vi "Sound Play Tone.vi"(5 "device ID":u32, 6 "stop":bool, 7 "Wait":bool=TRUE, 8 "error in":errorcluster, 9 "volume":dbl=100.0, 10 "sample duration (s)":dbl=0.25, 11 "frequency":dbl=440.0 format="%0.2p") -> (0 "error out":errorcluster, 4 "stopped":bool)   [LabVIEW 2018]
doc: "Plays a tone on an audio device.\n\nThe <b>wait</b> input causes this VI to block until the audio card has played all generated samples, so the execution time of the VI will be at least <b>sample duration(s)</b> long. Setting <b>wait</b> to false will cause the VI to return immediately; if used in an untimed loop, it will consume 100% resources. Set <b>wait</b> to true and use in an untimed loop to generate continuous output without overutilizing CPU resources.\n\nThis VI is written like an express VI: references and tasks are opened on first call, sound is output on every call (unless output fails), and the stop input closes all tasks. Use the stopped output to wire into the conditional terminal of a loop."
uses:
  <vilib>/sound2/lvsound2.llb/Sampling Mode.ctl
  <vilib>/sound2/lvsound2.llb/Sound Output Set Volume (Single).vi
  <vilib>/sound2/lvsound2.llb/Sound Output Write (DBL Single).vi
  <vilib>/measure/NI_MABase.lvlib
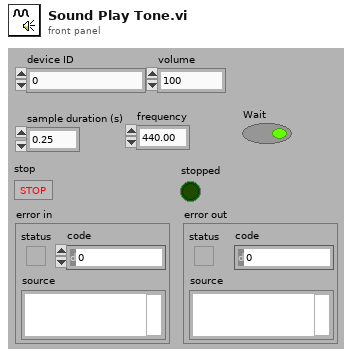
[diagram p1: front panel]
types:
  T1 = typedef "Sampling Mode.ctl" = i32
  T2 = cluster{"Sample Rate":dbl, "nChannels":i32, "Bits per Channel":i32}
  T3 = typedef "Sound Output Task ID.ctl" = u32
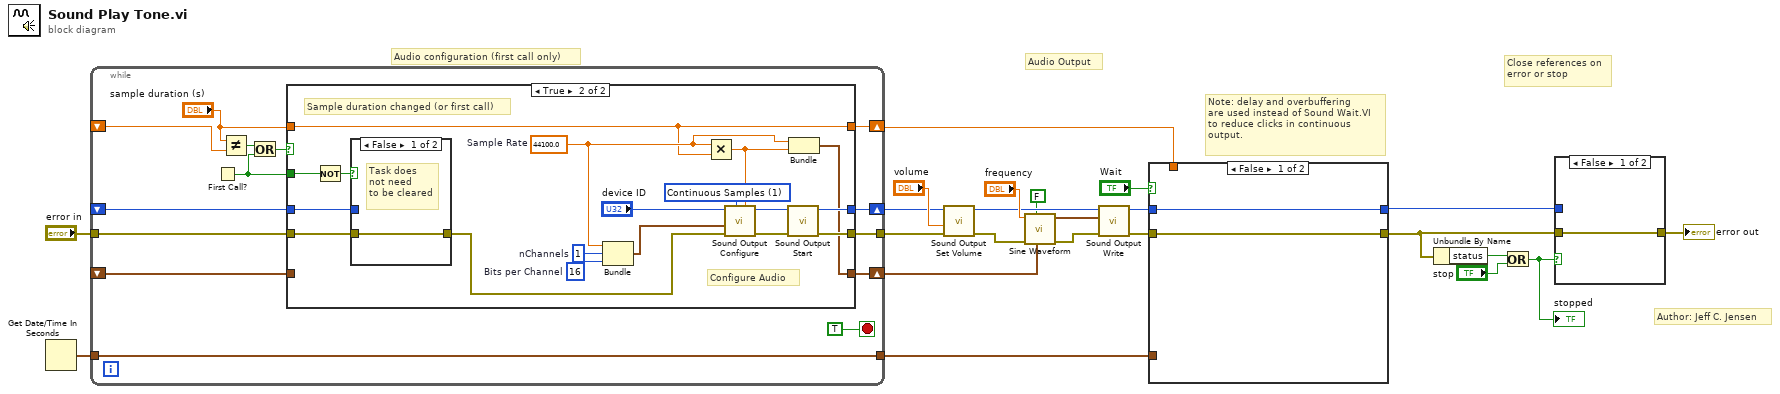
[diagram p0: block diagram]
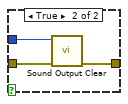
[diagram p2: hidden frame]
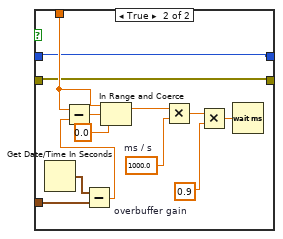
[diagram p3: hidden frame]
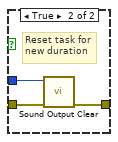
[diagram p5: hidden frame]
diagram:
  # "Note: delay and overbuffering\nare used instead of Sound Wait.VI\nto reduce clicks in continuous\noutput."
  # "Close references on\nerror or stop"
  # "Audio Output"
  # "Author: Jeff C. Jensen"
  # "Audio configuration (first call only)"
  n1 = Get Date/Time In Seconds() -> (seconds since 1Jan1904=w3:timestamp)
  n2 = while {
    tunnel: "error in" -> [w33]
    tunnel: [w37] -> w22
    shift-right: [w35] -> w5
    shift-left: _ -> [w32]
    shift-right: [w34] -> w4
    shift-left: _ -> [w31]
    shift-right: [w30] -> w1
    shift-left: _ -> [w26]
    tunnel: [w24] -> w2
    tunnel: w3 -> [w24]
    stop <- TRUE stop-if-true
    n3 = First Call?() -> (First Call?: T/F=w27:bool)
    n4 = Not Equal?(x="sample duration (s)", y=w26) -> (x != y?=w28:bool)
    n5 = Or(x=w28, y=w27) -> (x .or. y?=w29:bool)
    n6 = case shown="True" w29 {
      tunnel: [w39 w59] -> w37
      tunnel: [w41 w58] -> w35
      tunnel: [w40 w49] -> w34
      tunnel: w33 -> [w39 w46]
      tunnel: w32 -> [w41 w47]
      tunnel: w31 -> [w40 _]
      tunnel: [w38 w42] -> w30
      tunnel: "sample duration (s)" -> [w38 w42]
      tunnel: w27 -> [_ w43]
      frame False {
        # "Audio task already configured."
      }
      frame True {
        w53 = T1 1 items=["Finite Samples", "Continuous Samples"] ("sample mode")
        w48 = 44100.0  # Sample Rate
        w54 = 16  # Bits per Channel
        w55 = 1  # nChannels
        # "Sample duration changed (or first call)"
        # "Configure Audio"
        n7 = Not(x=w43) -> (.not. x?=w45:bool)
        n8 = case shown="False" w45 {
          tunnel: w47 -> [_ w63]
          tunnel: w46 -> [w60 w62]
          tunnel: [w60 w61] -> w44
          frame False {
            # "Task does\nnot need\nto be cleared"
          }
          frame True {
            # "Reset task for\nnew duration"
            n9 = call <vilib>:"Sound Output Clear.vi"("error in (no error)"=w62, "task ID"=w63) -> ("error out"=w61:errorcluster)  [unwired: 9 in]
          }
        }
        n10 = Bundle("Sample Rate"=w48, "nChannels"=w55, "Bits per Channel"=w54) -> (w56:T2)  [unwired: 1 in]
        n11 = Multiply(x=w48, y=w42) -> (x*y=w52:dbl)
        n12 = call <vilib>:"Sound Output Configure.vi"("number of samples/ch"=w52, "sample mode"=w53, "error in (no error)"=w44, "sound format"=w56, "device ID"="device ID") -> ("error out"=w51:errorcluster, "task ID"=w50:T3)  [unwired: 5 in]
        n13 = call <vilib>:"Sound Output Start.vi"("error in (no error)"=w51, "task ID"=w50) -> ("error out"=w59:errorcluster, "task ID out"=w58:T3)  [unwired: 8 in]
        n14 = Bundle("Sample Rate"=w48, w52) -> (w49:cluster{"Sample Rate":dbl, dbl})  [unwired: 1 in]
      }
    }
  }
  n15 = call-poly <vilib>:"Sound Output Set Volume.vi"("error in (no error)"=w22, "volume"="volume", "task ID"=w5) -> ("error out"=w20:errorcluster, "task ID out"=w18:T3)  [unwired: 7 in]
  n16 = call <vilib>:"Sine Waveform.vi"("sampling info"=w4, "reset signal"=FALSE, "error in (no error)"=w20, "frequency"="frequency") -> ("error out"=w17:errorcluster, "signal out"=w16:waveform(dbl))  [unwired: 6 in]
  n17 = call-poly <vilib>:"Sound Output Write.vi"("error in (no error)"=w17, "data"=w16, "task ID"=w18) -> ("error out"=w14:errorcluster, "task ID out"=w15:T3)  [unwired: 7 in]
  n18 = case shown="False" "Wait" {
    tunnel: w15 -> [w65 w70]
    tunnel: w14 -> [w64 w69]
    tunnel: [w64 w69] -> w8
    tunnel: [w65 w70] -> w7
    tunnel: w1 -> [_ w71]
    tunnel: w2 -> [_ w78]
    frame False {
    }
    frame True {
      w68 = 0.9  # overbuffer gain
      w72 = 1000.0  # ms / s
      n19 = Get Date/Time In Seconds() -> (seconds since 1Jan1904=w77:timestamp)
      n20 = Subtract(x=w77, y=w78) -> (x-y=w74:dbl)
      n21 = Subtract(x=w71, y=w74) -> (x-y=w76:dbl)
      n22 = In Range and Coerce(upper limit=w71, x=w76, lower limit=0.0) -> (coerced(x)=w73:dbl)  [unwired: 1 out]
      n23 = Multiply(x=w73, y=w72) -> (x*y=w67:dbl)
      n24 = Multiply(x=w67, y=w68) -> (x*y=w66:dbl)
      n25 = Wait (ms)(milliseconds to wait=w66) -> ()  [unwired: 1 out]
    }
  }
  n26 = Unbundle By Name(w8) -> ("status"=w11:bool)
  n27 = Or(x=w11, y="stop") -> (x .or. y?=w9:bool)
  "stopped" <- w9
  n28 = case shown="False" w9 {
    tunnel: w8 -> [w79 w82]
    tunnel: w7 -> [_ w80]
    tunnel: [w79 w81] -> w6
    frame False {
    }
    frame True {
      n29 = call <vilib>:"Sound Output Clear.vi"("error in (no error)"=w82, "task ID"=w80) -> ("error out"=w81:errorcluster)  [unwired: 9 in]
    }
  }
  "error out" <- w6
